vi "Http_Test.vi"() -> ()   [LabVIEW 2012]
uses:
  Libs/Http/Form.ctl
  Libs/Http/Method.ctl
  Libs/Http/Http.lvclass
panel:
  out "数组":string[][](array[string])
  in  "±í†Î":T1
  in  "Url":string="http://127.0.0.1/ESDCheck_PHPScript/DataInOut/"
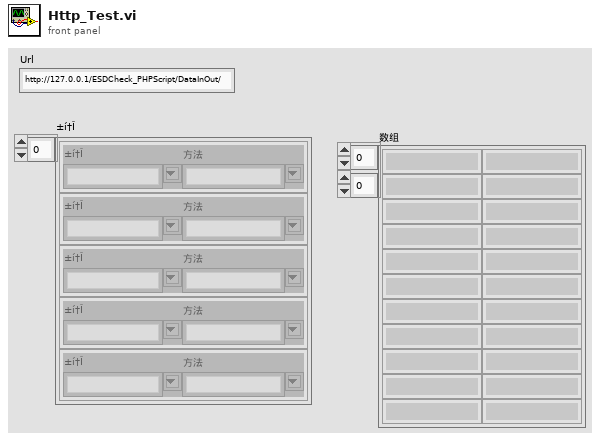
[diagram p1: front panel]
types:
  T1 = typedef "Http.lvclass/Form.ctl" = cluster{"±í†Î":string, "方法":T2}[]
  T2 = typedef "Http.lvclass/Method.ctl" = string
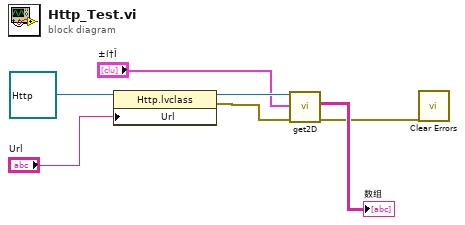
[diagram p0: block diagram]
diagram:
  n1 = property class="Http.lvclass"(reference=refnum<class "Http.lvclass"> refnum ("HttpClient.lvclass"), "Url"="Url") -> (reference out=w5:refnum<class "Http.lvclass">, error out=w4:errorcluster)  [unwired: 1 in]
  n2 = call-dynamic "get2D.vi"("error in (no error)"=w4, "±í†Î”µ“þ"="±í†Î", "HttpClient 输入"=w5) -> ("error out"=w1:errorcluster, "数组"=→"数组":string[][])  [unwired: 6 in, 1 out]
  n3 = call <vilib>:"Clear Errors.vi"("error in (no error)"=w1) -> ()  [unwired: 6 in, 1 out]
